vi "ClientSrv Log Server Error.vi"(0 "message (use cluster)":string, 11 "error (use message)":errorcluster) -> ()   [LabVIEW 2012]
doc: "Log a server-side error by sending it as a message to the \"errors\" task. This task asynchronously takes care of further processing. The error is first explained by accessing error code database if such was not done already."
uses:
  luaview/typedefs/t_LuaVIEW Task List Methods.ctl
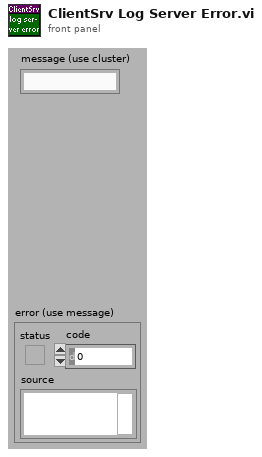
[diagram p1: front panel]
types:
  T1 = typedef "t_LuaVIEW Task List Methods.ctl" = enum16{"clear list", "add", "test", "remove", "get ref", "get task info", "get list", "get script info", "ongoing?", "resume", "pause", "stop", "confirm", "message"}
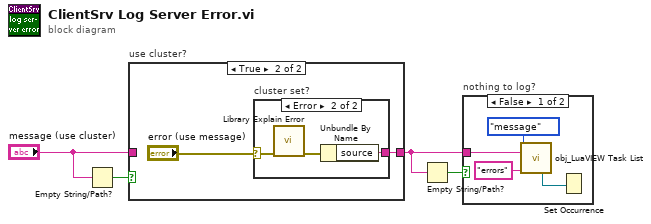
[diagram p0: block diagram]
diagram:
  n1 = Empty String/Path?(string/path="message (use cluster)") -> (empty?=w4:bool)
  n2 = case "use cluster?" shown="True" w4 {
    tunnel: [w5 w7] -> w2
    tunnel: "message (use cluster)" -> [w5 _]
    frame False {
    }
    frame True {
      n3 = case "cluster set?" shown="Error" "error (use message)" {
        selector: "error (use message)" -> [_ w8]
        tunnel: [_ w10] -> w7
        frame No Error {
        }
        frame Error {
          n4 = call "Library Explain Error.vi"("error in (no error)"=w8) -> ("explained error"=w9:errorcluster)  [unwired: 14 in]
          n5 = Unbundle By Name(w9) -> ("source"=w10:string)
        }
      }
    }
  }
  n6 = Empty String/Path?(string/path=w2) -> (empty?=w1:bool)
  n7 = case "nothing to log?" shown="False" w1 {
    tunnel: w2 -> [w12 _]
    frame False {
      n8 = call "obj_LuaVIEW Task List.vi"("method"=t_LuaVIEW_Task_List_Methods."message", "message"=w12, "task identifier"="errors") -> ("wakeup occurrence"=w11:refnum<k4>)  [unwired: 7 in, 5 out]
      n9 = Set Occurrence(w11) -> ()
    }
    frame True {
    }
  }
